vi "TraverseDoAllChannels.vi"(4 "Traverse Name":string="EnFlo Tunnel", 5 "Counters Reset?":bool, 6 "Matched Configurations all Channels In":T1[](array[typedef]) {"Static Drive Configuration"."Indexer Mode  (FSA)" items=["Incremental", "Absolute"]; "Static Drive Configuration"."Buffer at Stop (SSH)" items=["Clear buffer", "Save and Continue"]; "Static Drive Configuration"."Buffer at Limit (SSG)" items=["Clear buffer", "Save and Continue"]; "Static Drive Configuration"."RS232 Echo Control (SSA)" items=["Echo ON", "Echo OFF"]; "Static Drive Configuration"."Reference edge of Home (OSH)" items=["CW", "CCW"]; "Static Drive Configuration"."Encoder Z for Home (OSD)" items=["Don't use", "Enable"]; "Static Drive Configuration"."Home Switch Sense (OSC)" items=["Normally Open", "Normally Closed"]; "Static Drive Configuration"."Home Position (OSB)" items=["Anywhere in Switch", "Edge of Switch"]; "Static Drive Configuration"."Limit Switch Sense (OSA)" items=["Normally Closed", "Normally Open"]; "Static Drive Configuration"."Limit Disable (LD)" items=["Both Enabled", "CW Disabled", "CCW Disabled", "Both Disabled"]; "Static Drive Configuration"."Stall Detect (FSH)" items=["Disable", "Enable"]; "Static Drive Configuration"."OP2 in Deadband (FSG)" items=["Don't Use", "ACTIVATE"]; "Static Drive Configuration"."Stop on Trigger 3 (FSF)" items=["Ignore", "STOP!"]; "Static Drive Configuration"."Activate OP1 on stall (FSE)" items=["Do not Activate", "ACTIVATE!"]; "Static Drive Configuration"."Stop on Stall (FSD)" items=["Continue", "STOP"]; "Static Drive Configuration"."Position Maintenance (FSC)" items=["Disabled", "Enabled"]; "Static Drive Configuration"."Step Mode  (FSB)" items=["Motor", "Encoder"]; "Static Drive Configuration"."Encoder Resolution (ER)" min=1 max=50000; "Static Drive Configuration"."Dead Band Window (DW)" min=0 max=999999999; "Static Drive Configuration"."Dead Band (DB)" min=0 max=999999999; "Static Drive Configuration"."Correction Gain % (CG)" items=["n/a", "12.5", "25", "37.5", "50", "62.5", "75", "87.5", "100"]; "Channel Properties"."Current Pos" format="%.2f"; "Channel Properties"."Backlash/Eng units" format="%.2f"; "Channel Properties"."Pulses/rev" format="%.2f"; "Channel Properties"."Pos Tolerance" format="%.2f"; "Channel Properties"."Pulses/unit" format="%.2f"; "Channel Properties"."Acc. Min" format="%.2f"; "Channel Properties"."Acc. Max" format="%.2f"; "Channel Properties"."Vel. Min" format="%.2f"; "Channel Properties"."Vel. Max" format="%.2f"; "Channel Properties"."Acc. Default" format="%.2f"; "Channel Properties"."Vel. Default" format="%.2f"}, 7 "Current Pos In Eng units of all channels":dbl[](array[numeric]) format="%.2f", 8 "Position Steps":dbl[][](array[numeric]) format="%.2f", 9 "Mode":T4, 10 "Backlash Compensation?":bool, 11 "Current Pulses positions for all channels":dbl[](array[numeric])) -> (0 "Matched Configurations Out":T1[](array[typedef]) {"Static Drive Configuration"."Indexer Mode  (FSA)" items=["Incremental", "Absolute"]; "Static Drive Configuration"."Buffer at Stop (SSH)" items=["Clear buffer", "Save and Continue"]; "Static Drive Configuration"."Buffer at Limit (SSG)" items=["Clear buffer", "Save and Continue"]; "Static Drive Configuration"."RS232 Echo Control (SSA)" items=["Echo ON", "Echo OFF"]; "Static Drive Configuration"."Reference edge of Home (OSH)" items=["CW", "CCW"]; "Static Drive Configuration"."Encoder Z for Home (OSD)" items=["Don't use", "Enable"]; "Static Drive Configuration"."Home Switch Sense (OSC)" items=["Normally Open", "Normally Closed"]; "Static Drive Configuration"."Home Position (OSB)" items=["Anywhere in Switch", "Edge of Switch"]; "Static Drive Configuration"."Limit Switch Sense (OSA)" items=["Normally Closed", "Normally Open"]; "Static Drive Configuration"."Limit Disable (LD)" items=["Both Enabled", "CW Disabled", "CCW Disabled", "Both Disabled"]; "Static Drive Configuration"."Stall Detect (FSH)" items=["Disable", "Enable"]; "Static Drive Configuration"."OP2 in Deadband (FSG)" items=["Don't Use", "ACTIVATE"]; "Static Drive Configuration"."Stop on Trigger 3 (FSF)" items=["Ignore", "STOP!"]; "Static Drive Configuration"."Activate OP1 on stall (FSE)" items=["Do not Activate", "ACTIVATE!"]; "Static Drive Configuration"."Stop on Stall (FSD)" items=["Continue", "STOP"]; "Static Drive Configuration"."Position Maintenance (FSC)" items=["Disabled", "Enabled"]; "Static Drive Configuration"."Step Mode  (FSB)" items=["Motor", "Encoder"]; "Static Drive Configuration"."Encoder Resolution (ER)" min=1 max=50000; "Static Drive Configuration"."Dead Band Window (DW)" min=0 max=999999999; "Static Drive Configuration"."Dead Band (DB)" min=0 max=999999999; "Static Drive Configuration"."Correction Gain % (CG)" items=["n/a", "12.5", "25", "37.5", "50", "62.5", "75", "87.5", "100"]; "Channel Properties"."Current Pos" format="%.2f"; "Channel Properties"."Backlash/Eng units" format="%.2f"; "Channel Properties"."Pulses/rev" format="%.2f"; "Channel Properties"."Pos Tolerance" format="%.2f"; "Channel Properties"."Pulses/unit" format="%.2f"; "Channel Properties"."Acc. Min" format="%.2f"; "Channel Properties"."Acc. Max" format="%.2f"; "Channel Properties"."Vel. Min" format="%.2f"; "Channel Properties"."Vel. Max" format="%.2f"; "Channel Properties"."Acc. Default" format="%.2f"; "Channel Properties"."Vel. Default" format="%.2f"}, 1 "Error String":string, 3 "Achieved Pos In Eng units of all channels":dbl[](array[numeric]) format="%.2f")   [LabVIEW 2010]
uses:
  Anemometry/Anemometry Sub Vis/Gen Trav/Trav_mode.ctl
  ~subVIs/AxisConfigCluster.ctl
  ~subVIs/DriveProperties.ctl
  ~subVIs/DriveStaticConfig.ctl
  ~subVIs/DriveGotoCluster.ctl
  ~subVIs/DriveConfigGlobal.vi
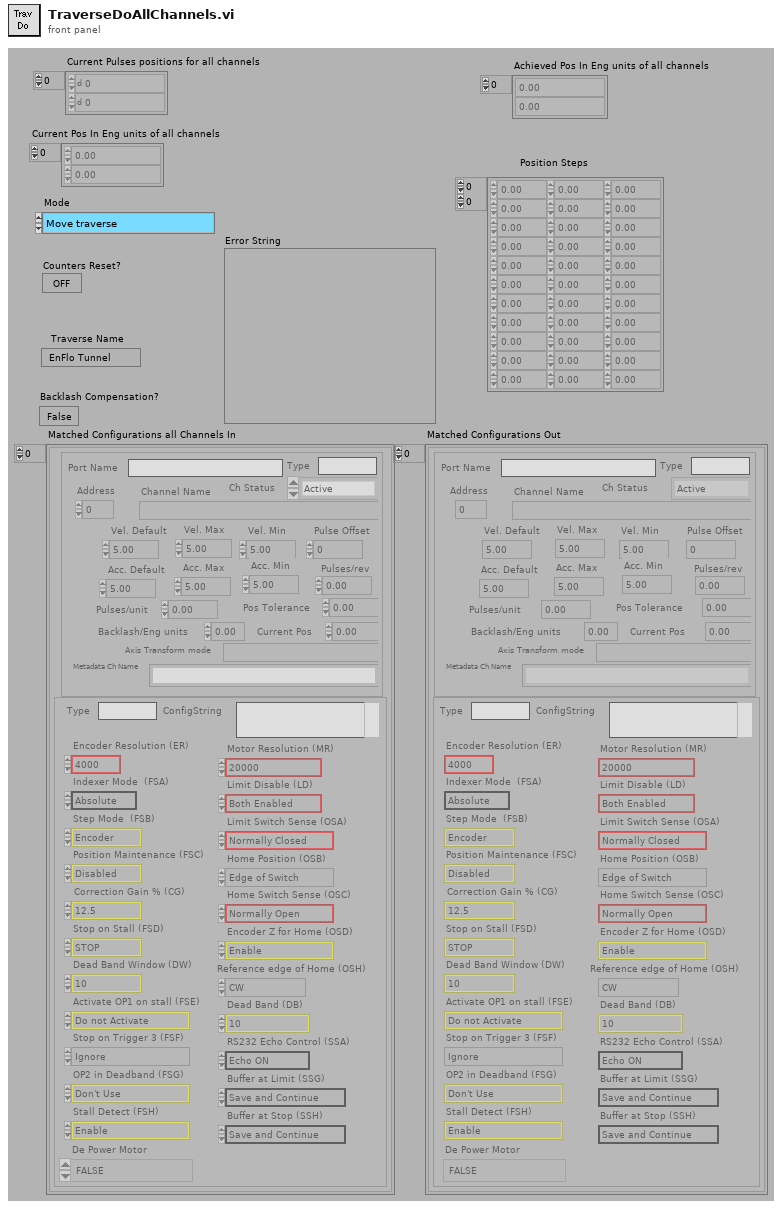
[diagram p1: front panel]
types:
  T1 = typedef "AxisConfigCluster.ctl" = cluster{"Channel Properties":T2, "Static Drive Configuration":T3}
  T2 = typedef "DriveProperties.ctl" = cluster{"Channel Name":string, "Vel. Default":dbl, "Acc. Default":dbl, "Vel. Max":dbl, "Vel. Min":dbl, "Acc. Max":dbl, "Acc. Min":dbl, "Pulses/unit":dbl, "Address":u8, "Pulse Offset":i32, "Pos Tolerance":dbl, "Pulses/rev":dbl, "Backlash/Eng units":dbl, "Current Pos":dbl, "Ch Status":enum16{"Active", "Offline", "Simulate"}, "Port Name":string, "Axis Transform mode":string, "Metadata Ch Name":string, "Type":string}
  T3 = typedef "DriveStaticConfig.ctl" = cluster{"Correction Gain % (CG)":u16, "Dead Band (DB)":i32, "Dead Band Window (DW)":i32, "Encoder Resolution (ER)":i32, "Step Mode  (FSB)":u16, "Position Maintenance (FSC)":u16, "Stop on Stall (FSD)":u16, "Activate OP1 on stall (FSE)":u16, "Stop on Trigger 3 (FSF)":u16, "OP2 in Deadband (FSG)":u16, "Stall Detect (FSH)":u16, "Limit Disable (LD)":u16, "Motor Resolution (MR)":enum16{"200", "400", "1000", "2000", "4000", "5000", "10000", "12800", "18000", "20000", "21600", "25000", "25400", "25600", "36000", "50000", "278528", "425984", "507904", "614400", "655360", "819200", "1024000"}, "Limit Switch Sense (OSA)":u16, "Home Position (OSB)":u16, "Home Switch Sense (OSC)":u16, "Encoder Z for Home (OSD)":u16, "Reference edge of Home (OSH)":u16, "RS232 Echo Control (SSA)":u16, "Buffer at Limit (SSG)":u16, "Buffer at Stop (SSH)":u16, "Indexer Mode  (FSA)":u16, "Type":string, "ConfigString":string, "De Power Motor":enum16{"TRUE", "FALSE"}}
  T4 = typedef "Trav_mode.ctl" = enum16{"Move traverse", "Read traverse position", "Teach Position"}
  T5 = enum16{"Load setup from excel file", "Save setup to excel file"}
  T6 = typedef "DriveGotoCluster.ctl" = cluster{"Channel name":string, "Go To Position":dbl}
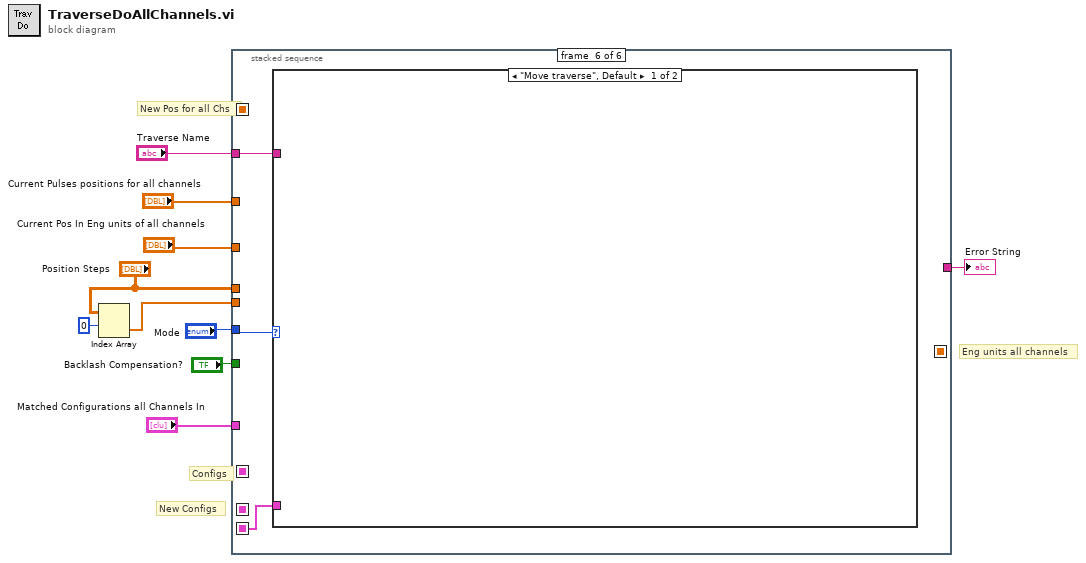
[diagram p0: block diagram]
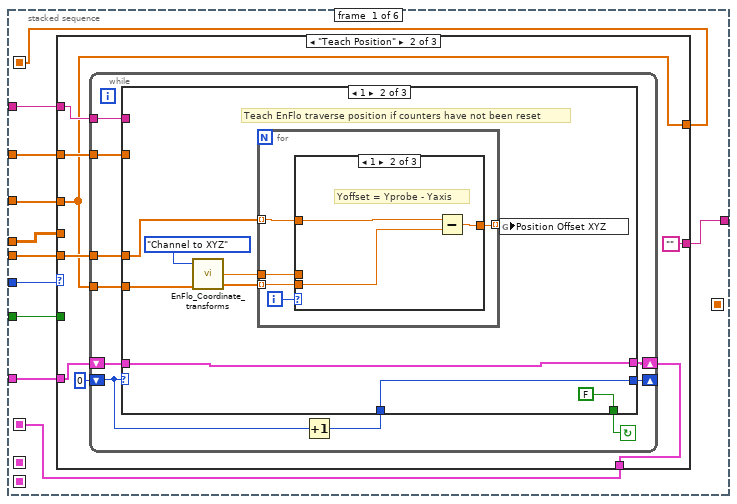
[diagram p2: hidden frame]
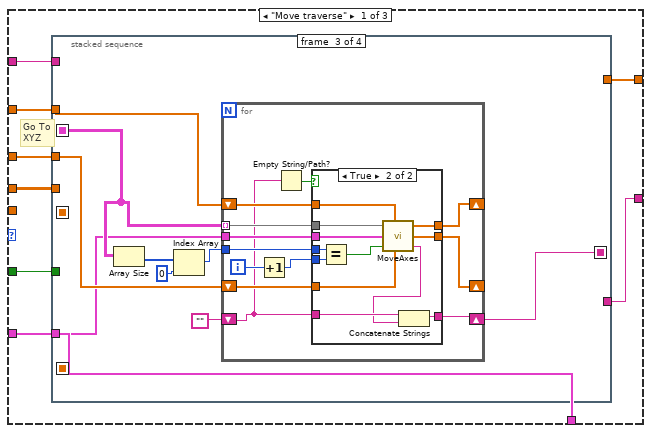
[diagram p3: hidden frame]
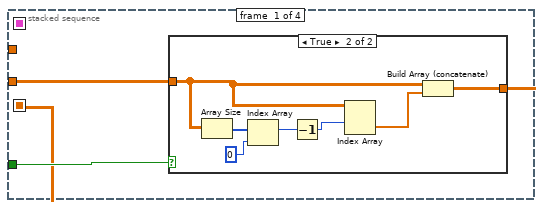
[diagram p4: hidden frame]
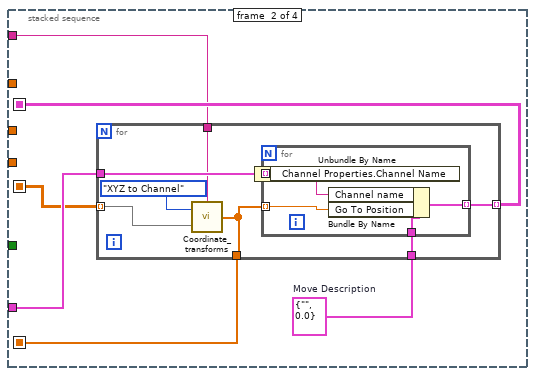
[diagram p6: hidden frame]
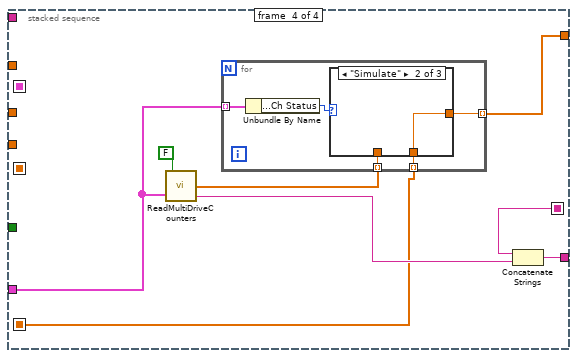
[diagram p8: hidden frame]
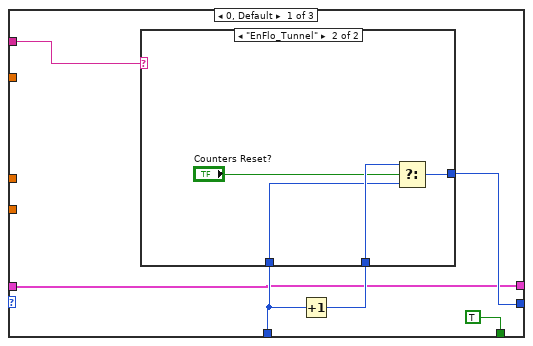
[diagram p11: hidden frame]
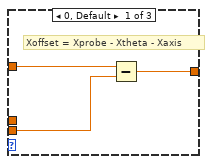
[diagram p13: hidden frame]
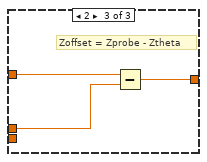
[diagram p14: hidden frame]
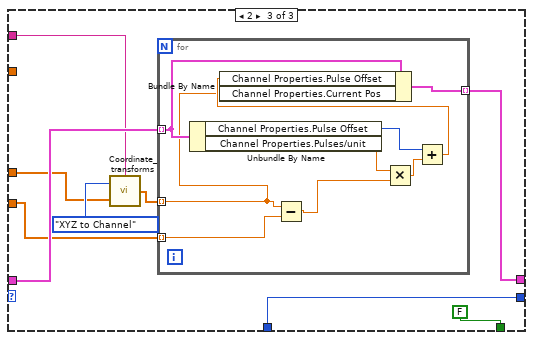
[diagram p15: hidden frame]
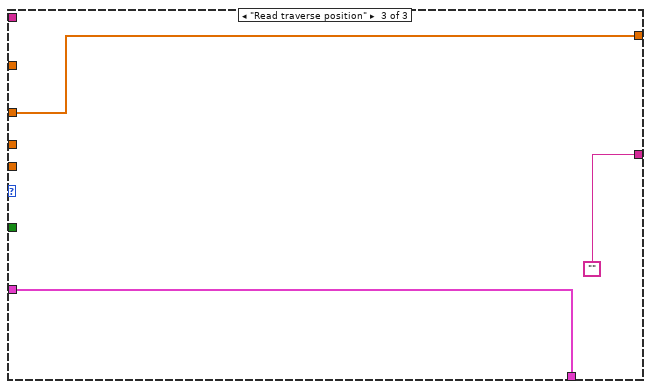
[diagram p16: hidden frame]
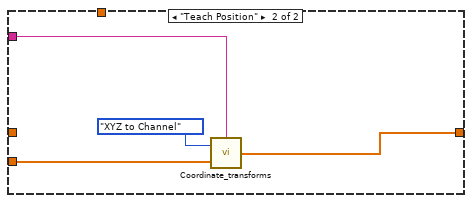
[diagram p18: hidden frame]
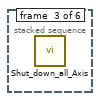
[diagram p19: hidden frame]
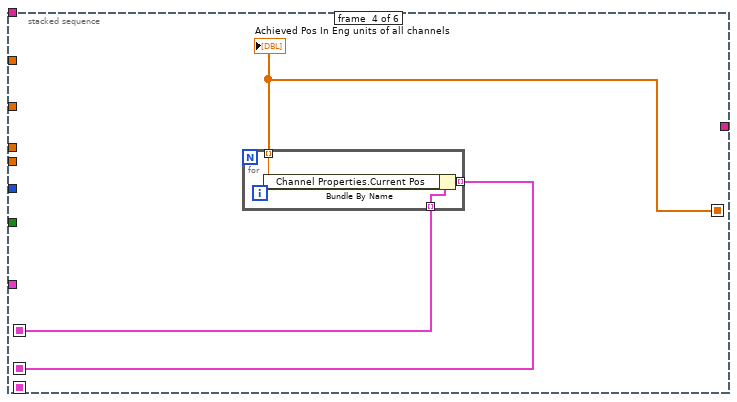
[diagram p20: hidden frame]
diagram:
  # "New Pos for all Chs"
  # "Eng units all channels"
  # "New Configs"
  # "Configs"
  n1 = Index Array(array="Position Steps", index (row)=0 ("Index")) -> (element=w1:dbl[])  [unwired: 1 in]
  n2 = stacked-sequence {
    seq-local: [_ w187 _ _ _ _] -> [_ _ _ w195 _ _]
    seq-local: [w20 _ _ _ _ _] -> [_ _ _ w197 _ _]
    seq-local: [_ _ _ w196 _ _] -> [_ _ _ _ w203 _]
    seq-local: [w11 _ _ _ _ _] -> [_ w184 _ _ _ _]
    seq-local: [_ _ _ _ w201 _] -> [_ _ _ _ _ w206]
    tunnel: "Mode" -> [w21 w188 _ _ _ w207]
    tunnel: "Current Pos In Eng units of all channels" -> [w18 w189 _ _ _ _]
    tunnel: "Matched Configurations all Channels In" -> [w19 _ _ _ _ _]
    tunnel: "Current Pulses positions for all channels" -> [w17 _ _ _ _ _]
    tunnel: [w16 _ _ _ _ _] -> w6
    tunnel: "Traverse Name" -> [w15 w186 _ _ w202 w205]
    tunnel: "Position Steps" -> [w14 _ _ _ _ _]
    tunnel: "Backlash Compensation?" -> [w13 _ _ _ _ _]
    tunnel: w1 -> [w12 w185 _ _ _ _]
    frame #0 {
      n3 = case shown="\"Teach Position\"" w21 {
        tunnel: [w29 w114 w183] -> w20
        tunnel: w19 -> [w29 w115 w183]
        tunnel: w18 -> [w27 w111 w181]
        tunnel: w17 -> [w28 w116 _]
        tunnel: [w26 "" ""] -> w16
        tunnel: w15 -> [w24 w117 _]
        tunnel: w14 -> [w25 _ _]
        tunnel: w13 -> [w23 _ _]
        tunnel: w12 -> [_ w112 _]
        tunnel: [w22 w111 w181] -> w11
        frame "Move traverse" {
          # "Go To\nXYZ"
          n4 = stacked-sequence {
            seq-local: [_ w44 _ _] -> [_ _ w61 _]
            seq-local: [w31 _ _ _] -> [_ w43 _ _]
            seq-local: [_ _ w59 _] -> [_ _ _ w101]
            seq-local: [_ w41 _ _] -> [_ _ _ w95]
            tunnel: w29 -> [_ w45 w60 w98]
            tunnel: w28 -> [_ _ w67 _]
            tunnel: w27 -> [_ _ w66 _]
            tunnel: [_ _ _ w99] -> w26
            tunnel: w25 -> [w30 _ _ _]
            tunnel: w24 -> [_ w42 _ _]
            tunnel: w23 -> [w32 _ _ _]
            tunnel: [_ _ _ w97] -> w22
            frame #0 {
              n5 = case shown="True" w32 {
                tunnel: w30 -> [w33 w35]
                tunnel: [w33 w34] -> w31
                frame False {
                }
                frame True {
                  n6 = Array Size(array=w35) -> (size(s)=w40:i32[])
                  n7 = Index Array(array=w40, index=0 ("Index")) -> (element=w38:i32)
                  n8 = Decrement(x=w38) -> (x-1=w37:i32)
                  n9 = Index Array(array=w35, index (row)=w37) -> (element=w36:dbl[])  [unwired: 1 in]
                  n10 = Build Array (concatenate)(w35, w36) -> (w34:dbl[][])
                }
              }
            }
            frame #1 {
              w46 = T6 {"Channel name"="", "Go To Position"=0.0}  # Move Description
              n11 = for {
                tunnel: w46 -> [w53]
                tunnel: w45 -> [w52]
                tunnel: [w51] -> w44 mode=indexing
                tunnel: w43 -> [w48] mode=indexing
                tunnel: w42 -> [w49]
                tunnel: [w47] -> w41
                n12 = call "Coordinate_transforms.vi"("Traverse Name"=w49, "Input"=w48, "Mode"=enum16{"XYZ to Channel", "Channel to XYZ"}."XYZ to Channel") -> ("Output"=w47:dbl[])
                n13 = for {
                  tunnel: w47 -> [w58] mode=indexing
                  tunnel: [w57] -> w51 mode=indexing
                  tunnel: w52 -> [w55] mode=indexing
                  tunnel: w53 -> [w54]
                  n14 = Unbundle By Name(w55) -> ("Channel Properties.Channel Name"=w56:string)
                  n15 = Bundle By Name(cluster=w54, "Channel name"=w56, "Go To Position"=w58) -> (w57:T6)
                }
              }
            }
            frame #2 {
              n16 = Array Size(array=w61) -> (size(s)=w64:i32[])
              n17 = Index Array(array=w64, index=0 ("Index")) -> (element=w62:i32)
              n18 = for {
                tunnel: w61 -> [w79] mode=indexing
                tunnel: w60 -> [w78]
                shift-right: [w75] -> _
                shift-left: w67 -> [w74]
                shift-right: [w76] -> _
                shift-left: w66 -> [w77]
                tunnel: w62 -> [w71]
                shift-right: [w70] -> w59
                shift-left: "" -> [w69]
                i -> [w73]
                n19 = Increment(x=w73) -> (x+1=w72:i32)
                n20 = Empty String/Path?(string/path=w69) -> (empty?=w68:bool)
                n21 = case shown="True" w68 {
                  tunnel: w79 -> [_ w94]
                  tunnel: w78 -> [_ w93]
                  tunnel: w77 -> [w81 w92]
                  tunnel: [w81 w91] -> w76
                  tunnel: [w82 w90] -> w75
                  tunnel: w74 -> [w82 w89]
                  tunnel: w72 -> [_ w88]
                  tunnel: w71 -> [_ w87]
                  tunnel: [w80 w84] -> w70
                  tunnel: w69 -> [w80 w86]
                  frame False {
                  }
                  frame True {
                    n22 = Equal?(x=w87, y=w88) -> (x = y?=w83:bool)
                    n23 = call "MoveAxes.vi"("GoTo Array (Eng units all channels)"=w94, "Current Pulses In"=w89, "Matched Configurations"=w93, "Final move"=w83, "Current Pos In"=w92) -> ("Current Pulses Out"=w90:dbl[], "Current Pos Out"=w91:dbl[], "Error String"=w85:string)
                    n24 = Concatenate Strings(w86, w85) -> (w84:string)
                  }
                }
              }
            }
            frame #3 {
              n25 = call "ReadMultiDriveCounters.vi"("Recheck if Moved?"=FALSE, "Matched Configurations"=w98) -> ("Eng units"=w96:dbl[], "Error String"=w100:string)  [unwired: 1 out]
              n26 = for {
                tunnel: w98 -> [w107] mode=indexing
                tunnel: [w105] -> w97 mode=indexing
                tunnel: w96 -> [w104] mode=indexing
                tunnel: w95 -> [w103] mode=indexing
                n27 = Unbundle By Name(w107) -> ("Channel Properties.Ch Status"=w106:enum16{"Active", "Offline", "Simulate"})
                n28 = case shown="\"Simulate\"" w106 {
                  tunnel: [w108 w109 w110] -> w105
                  tunnel: w104 -> [w108 _ w110]
                  tunnel: w103 -> [_ w109 _]
                  frame "Active" {
                  }
                  frame "Simulate" {
                  }
                  frame "Offline" {
                  }
                }
              }
              n29 = Concatenate Strings(w101, w100) -> (w99:string)
            }
          }
        }
        frame "Teach Position" {
          n30 = while {
            tunnel: w112 -> [w119]
            shift-left: w115 -> [w121]
            shift-right: [w120] -> w114
            tunnel: w111 -> [w122]
            tunnel: w116 -> [w123]
            tunnel: w117 -> [w124]
            shift-left: 0 -> [w128]
            shift-right: [w125] -> _
            stop <- w127 continue-if-true
            n31 = Increment(x=w128) -> (x+1=w126:i32)
            n32 = case shown="1" w128 {
              tunnel: [TRUE FALSE FALSE] -> w127
              tunnel: w126 -> [w131 w142 w171]
              tunnel: [w132 w142 w171] -> w125
              tunnel: w124 -> [w133 _ w164]
              tunnel: w123 -> [_ _ _]
              tunnel: w122 -> [_ w143 w165]
              tunnel: w121 -> [w129 w141 w169]
              tunnel: [w129 w141 w168] -> w120
              tunnel: w119 -> [_ w140 w163]
              frame 0, Default {
                n33 = Increment(x=w131) -> (x+1=w130:i32)
                n34 = case shown="\"EnFlo_Tunnel\"" w133 {
                  tunnel: [w135 w139] -> w132
                  tunnel: w131 -> [_ w137]
                  tunnel: w130 -> [w135 w138]
                  frame "A_Tunnel", Default {
                  }
                  frame "EnFlo_Tunnel" {
                    n35 = Select(t=w138, s="Counters Reset?", f=w137) -> (s? t:f=w139:i32)
                  }
                }
              }
              frame 1 {
                # "Teach EnFlo traverse position if counters have not been reset"
                n36 = call "EnFlo_Coordinate_transforms.vi"("Input"=w143, "Mode"=enum16{"XYZ to Channel", "Channel to XYZ"}."Channel to XYZ") -> ("Output"=w146:dbl[], "Z theta"=w145:dbl)  [unwired: 2 out]
                n37 = for {
                  tunnel: w140 -> [w152] mode=indexing
                  tunnel: w146 -> [w151] mode=indexing
                  tunnel: [w150] -> w147 mode=indexing
                  tunnel: w145 -> [w149]
                  i -> [w153]
                  n38 = case shown="1" w153 {
                    tunnel: w152 -> [w156 w159 w162]
                    tunnel: w151 -> [w155 w158 _]
                    tunnel: [w154 w157 w160] -> w150
                    tunnel: w149 -> [_ _ w161]
                    frame 0, Default {
                      # "Xoffset = Xprobe - Xtheta - Xaxis"
                      n39 = Subtract(x=w156, y=w155) -> (x-y=w154:dbl)
                    }
                    frame 1 {
                      # "Yoffset = Yprobe - Yaxis"
                      n40 = Subtract(x=w159, y=w158) -> (x-y=w157:dbl)
                    }
                    frame 2 {
                      # "Zoffset = Zprobe - Ztheta"
                      n41 = Subtract(x=w162, y=w161) -> (x-y=w160:dbl)
                    }
                  }
                }
                n42 = global write "DriveConfigGlobal.vi" "Position Offset XYZ"(w147) -> ()
              }
              frame 2 {
                n43 = call "Coordinate_transforms.vi"("Traverse Name"=w164, "Input"=w163, "Mode"=enum16{"XYZ to Channel", "Channel to XYZ"}."XYZ to Channel") -> ("Output"=w166:dbl[])
                n44 = for {
                  tunnel: w169 -> [w180] mode=indexing
                  tunnel: [w178] -> w168 mode=indexing
                  tunnel: w165 -> [w176] mode=indexing
                  tunnel: w166 -> [w172] mode=indexing
                  n45 = Unbundle By Name(w180) -> ("Channel Properties.Pulse Offset"=w177:i32, "Channel Properties.Pulses/unit"=w175:dbl)
                  n46 = Subtract(x=w172, y=w176) -> (x-y=w173:dbl)
                  n47 = Multiply(x=w175, y=w173) -> (x*y=w174:dbl)
                  n48 = Add(x=w177, y=w174) -> (x+y=w179:dbl)
                  n49 = Bundle By Name(cluster=w180, "Channel Properties.Pulse Offset"=w179, "Channel Properties.Current Pos"=w172) -> (w178:T1)
                }
              }
            }
          }
        }
        frame "Read traverse position" {
        }
      }
    }
    frame #1 {
      # "Eng units all channels"
      n50 = case shown="\"Move traverse\", Default" w188 {
        tunnel: w189 -> [_ _]
        tunnel: [w190 w193] -> w187
        tunnel: w186 -> [_ w192]
        tunnel: w185 -> [_ w191]
        tunnel: w184 -> [w190 _]
        frame "Move traverse", Default {
        }
        frame "Teach Position" {
          n51 = call "Coordinate_transforms.vi"("Traverse Name"=w192, "Input"=w191, "Mode"=enum16{"XYZ to Channel", "Channel to XYZ"}."XYZ to Channel") -> ("Output"=w193:dbl[])
        }
      }
    }
    frame #2 {
      n52 = call "Shut_down_all_Axis.vi"() -> ()  [unwired: 1 out]
    }
    frame #3 {
      n53 = for {
        tunnel: [w200] -> w196 mode=indexing
        tunnel: w197 -> [w199] mode=indexing
        tunnel: w195 -> [w198] mode=indexing
        n54 = Bundle By Name(cluster=w199, "Channel Properties.Current Pos"=w198) -> (w200:T1)
      }
      "Achieved Pos In Eng units of all channels" <- w195
    }
    frame #4 {
      n55 = call "Read_Write_Trav_position.vi"("Matched Configurations In"=w203, "Mode"=T5."Save setup to excel file", "Traverse Name"=w202) -> ("Matched Configurations Out"=w201:T1[])  [unwired: 1 out]
      "Matched Configurations Out" <- w201
    }
    frame #5 {
      n56 = case shown="\"Move traverse\", Default" w207 {
        tunnel: w206 -> [_ w209]
        tunnel: w205 -> [_ w208]
        frame "Move traverse", Default {
        }
        frame "Teach Position" {
          n57 = stacked-sequence {
            tunnel: w209 -> [w212 _]
            tunnel: w208 -> [_ w222]
            frame #0 {
              n58 = global read "DriveConfigGlobal.vi" "Configurations"() -> (w211:T1[])
              n59 = for {
                tunnel: w211 -> [w221] mode=indexing
                tunnel: [w220] -> w213 mode=indexing
                n60 = Unbundle By Name(w221) -> ("Channel Properties.Channel Name"=w220:string)
              }
              n61 = for {
                tunnel: w213 -> [w219]
                tunnel: w212 -> [w214] mode=indexing
                shift-right: [w216] -> w210
                shift-left: w211 -> [w217]
                n62 = Unbundle By Name(w214) -> ("Channel Properties.Channel Name"=w218:string)
                n63 = Search 1D Array(1D array=w219, element=w218) -> (index of element=w215:i32)  [unwired: 1 out]
                n64 = Replace Array Subset(array=w217, new element=w214, index=w215) -> (w216:T1[])
              }
              n65 = global write "DriveConfigGlobal.vi" "Configurations"(w210) -> ()
            }
            frame #1 {
              n66 = call "Read_Write_Trav_Config.vi"("Traverse Name"=w222, "Mode"=T5."Save setup to excel file") -> ()  [unwired: 1 out]
            }
          }
        }
      }
    }
  }
  "Error String" <- w6
